vi "Alternate_Row_Color.vi"(7 "error in":errorcluster, 9 "State":T1, 10 "MCListbox Refnum in":refnum<vi>) -> (0 "error out":errorcluster, 3 "MCListbox Refnum out":refnum<vi>)   [LabVIEW 2012, in "ListBox_XControl.xctl"]
doc: "Perform alternate row colouring on the MC listbox to the number of rows visible or the number or rows of item names, whichever is larger\n(uses Xcontrol properties \"Alternating BG Color\" and \"Alternating BC Text Color\")"
uses:
  ListBox_XControl.xctl
  ListBox_State.ctl
  Order Type Def.ctl
  Value Filters.ctl
  <vilib>/Utility/miscctls.llb/LVRowAndColumnTypeDef.ctl
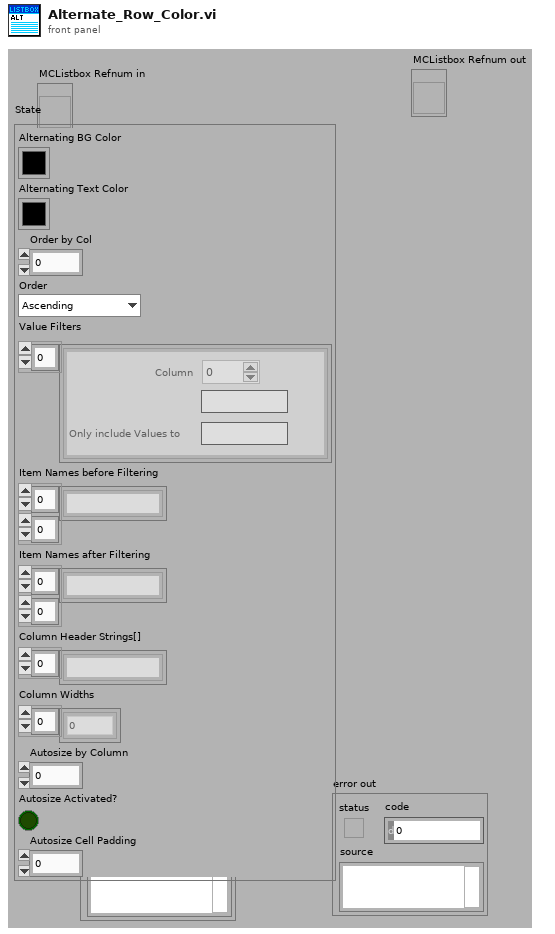
[diagram p1: front panel]
types:
  T1 = typedef "ListBox_XControl.xctl/ListBox_State.ctl" = cluster{"Alternating BG Color":u32, "Alternating Text Color":u32, "Order by Col":i32, "Order":T2, "Value Filters":T3, "Item Names before Filtering":string[][], "Item Names after Filtering":string[][], "Column Header Strings[]":string[], "Column Widths":u32[], "Autosize by Column":i32, "Autosize Activated?":bool, "Autosize Cell Padding":u32}
  T2 = typedef "ListBox_XControl.xctl/Order Type Def.ctl" = enum16{"Ascending", "Descending", "Off"}
  T3 = typedef "ListBox_XControl.xctl/Value Filters.ctl" = cluster{"Column":i32, "Only include Values From":string, "Only include Values to":string}[]
  T4 = typedef "LVRowAndColumnTypeDef.ctl" = cluster{"Row":i32, "Column":i32}
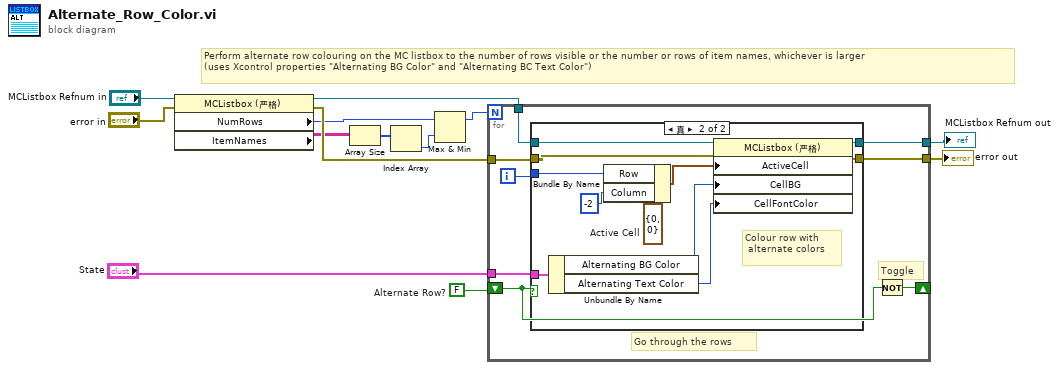
[diagram p0: block diagram]
diagram:
  w13 = FALSE  # Alternate Row?
  # "Perform alternate row colouring on the MC listbox to the number of rows visible or the number or rows of item names, whichever is larger\n(uses Xcontrol properties \"Alternating BG Color\" and \"Alternating BC Text Color\")"
  n1 = property on="Property Node" class="MCListbox (严格)"(reference="MCListbox Refnum in", error in="error in") -> (reference out=w3:refnum<vi>, error out=w10:errorcluster, "NumRows"=w7:u32, "ItemNames"=w5:string[][])
  n2 = Array Size(array=w5) -> (size(s)=w6:i32[])
  n3 = Index Array(array=w6) -> (element=w8:i32)  [unwired: 1 in]
  n4 = Max & Min(x=w7, y=w8) -> (max(x,y)=w9:u32)  [unwired: 1 out]
  n5 = for {
    N: w9 -> [_]
    tunnel: "State" -> [w14]
    tunnel: w10 -> [w20]
    tunnel: [w19] -> w11
    shift-right: [w17] -> _
    shift-left: w13 -> [w18]
    tunnel: w3 -> [w16]
    tunnel: [w15] -> w2
    i -> [w21]
    # "Go through the rows"
    # "Toggle"
    n6 = case shown="真" w18 {
      tunnel: w14 -> [_ w34]
      tunnel: w21 -> [_ w32]
      tunnel: w20 -> [w23 w30]
      tunnel: [w23 w29] -> w19
      tunnel: w16 -> [w22 w25]
      tunnel: [w22 w24] -> w15
      frame False {
        # "Colour row normally"
      }
      frame True {
        w33 = T4 {"Row"=0, "Column"=0}  # Active Cell
        # "Colour row with\n alternate colors"
        n7 = Unbundle By Name(w34) -> ("Alternating BG Color"=w27:u32, "Alternating Text Color"=w26:u32)
        n8 = Bundle By Name(cluster=w33, "Row"=w32, "Column"=-2) -> (w28:T4)
        n9 = property on="Property Node" class="MCListbox (严格)"(reference=w25, error in=w30, "ActiveCell"=w28, "CellBG"=w27, "CellFontColor"=w26) -> (reference out=w24:refnum<vi>, error out=w29:errorcluster)
      }
    }
    n10 = Not(x=w18) -> (.not. x?=w17:bool)
  }
  "error out" <- w11
  "MCListbox Refnum out" <- w2
